vi "Decimate and Interpolate (single).vi"(8 "error in (no error)":errorcluster, 10 "Configure":T1={"X Low"=0.05, "X High"=0.5, "X Step"=0.01, "fake point value"=0.05} {"fake point value" format="%#_6p"; "X Step" format="%#_6p"; "X High" format="%#_6p"; "X Low" format="%#_6p"}, 11 "XY-data in":cluster{"X-array":dbl[], "Y-array":dbl[]}) -> (0 "error out":errorcluster, 3 "XY-data out":cluster{"X-array":dbl[], "Y-array":dbl[]} {"Y-array" format="%.2p"; "X-array" format="%.2p"})   [LabVIEW 2016, in "xy_utilities.lvlib"]
uses:
  xy_utilities.lvlib
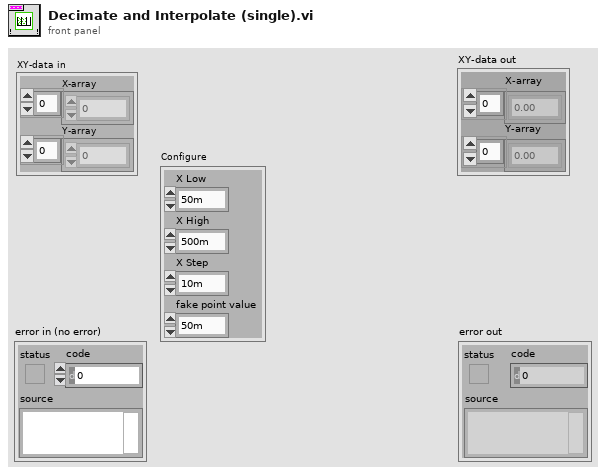
[diagram p1: front panel]
types:
  T1 = cluster{"X Low":dbl, "X High":dbl, "X Step":dbl, "fake point value":dbl}
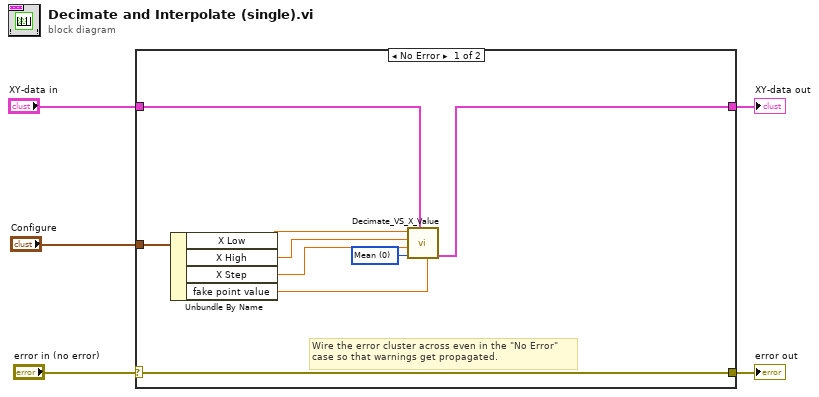
[diagram p0: block diagram]
diagram:
  n1 = case shown="No Error" "error in (no error)" {
    selector: "error in (no error)" -> [w14 w16]
    tunnel: [w14 w16] -> w4
    tunnel: "XY-data in" -> [w7 w15]
    tunnel: [w6 w15] -> w2
    tunnel: "Configure" -> [w12 _]
    frame No Error {
      w13 = u16 0 items=["Mean", "Max", "Min", "Sigma", "Median"] ("Method")
      # "Wire the error cluster across even in the \"No Error\"\ncase so that warnings get propagated."
      n2 = Unbundle By Name(w12) -> ("X Low"=w11:dbl, "X High"=w10:dbl, "X Step"=w9:dbl, "fake point value"=w8:dbl)
      n3 = call <userlib>:"Decimate_VS_X_Value.vi"("fake point value"=w8, "XY Graph kind 1"=w7, "Method"=w13, "X Step"=w9, "X High"=w10, "X Low"=w11) -> ("Interpreted"=w6:cluster{dbl[], dbl[]})  [unwired: 4 in, 1 out]
    }
    frame Error {
    }
  }
  "error out" <- w4
  "XY-data out" <- w2
